vi "Counter_Straight_MotorControl_r1 (SubVI).vi"(6 "Goal Y Coord":dbl, 9 "Goal X Coord":dbl, 10 "Current Y Pos":dbl, 11 "Current X Pos":dbl) -> (3 "Numeric out":dbl)   [LabVIEW 2015]
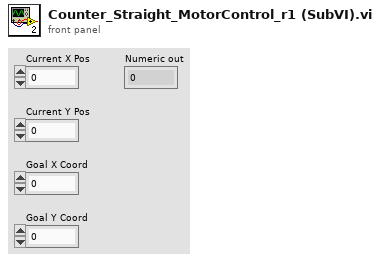
[diagram p1: front panel]
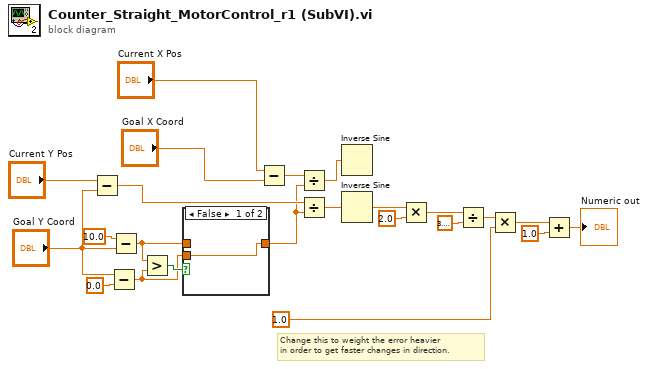
[diagram p0: block diagram]
diagram:
  # "Change this to weight the error heavier\nin order to get faster changes in direction."
  n1 = Subtract(x="Current Y Pos", y="Goal Y Coord") -> (x-y=w12:dbl)
  n2 = Subtract(x="Goal Y Coord", y=0.0 ("x")) -> (x-y=w2:dbl)
  n3 = Subtract(x=10.0, y="Goal Y Coord") -> (x-y=w3:dbl)
  n4 = Greater?(x=w3, y=w2) -> (0:w4:bool)
  n5 = case shown="False" w4 {
    tunnel: w3 -> [_ w25]
    tunnel: [w24 w25] -> w1
    tunnel: w2 -> [w24 _]
    frame False {
    }
    frame True {
    }
  }
  n6 = Subtract(x="Current X Pos", y="Goal X Coord") -> (x-y=w11:dbl)
  n7 = Divide(x=w11, y=w1) -> (x/y=w13:dbl)
  n8 = Divide(x=w12, y=w1) -> (x/y=w14:dbl)
  n9 = Inverse Sine(1:w13) -> ()  [unwired: 1 out]
  n10 = Inverse Sine(1:w14) -> (0:w15:dbl)
  n11 = Multiply(x=w15, y=2.0) -> (x*y=w17:dbl)
  n12 = Divide(x=w17, y=3.141592653589793) -> (x/y=w20:dbl)
  n13 = Multiply(x=w20, y=1.0) -> (x*y=w21:dbl)
  n14 = Add(x=w21, y=1.0) -> (x+y=→"Numeric out":dbl)
